vi "IMAQ-RGBtoIntensity.vi"(1 "Blue 2D Array":dbl[][](array[numeric]), 2 "Green 2D Array":dbl[][](array[numeric]), 3 "Red 2D Array":dbl[][](array[numeric])) -> (0 "Intensity 2D Array":dbl[][](array[numeric]))   [LabVIEW 2010]
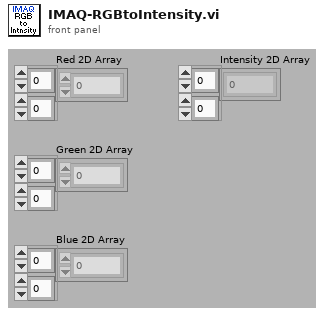
[diagram p1: front panel]
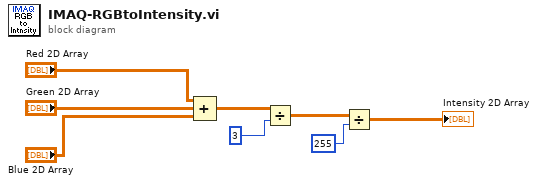
[diagram p0: block diagram]
diagram:
  n1 = Compound Arithmetic op=ADD("Red 2D Array", "Green 2D Array", "Blue 2D Array") -> (w4:dbl[][])
  n2 = Divide(x=w4, y=3) -> (x/y=w3:dbl[][])
  n3 = Divide(x=w3, y=255) -> (x/y=→"Intensity 2D Array":dbl[][])
